vi "Curva suporte.vi"(8 "error in (no error)":errorcluster, 11 "Dados SP":T1={"Condutor"={"Pc (N/m)"=0.0, "Mod.Young (N/m²)"=0.0, "Dil.Term.c (m/°C)"=0.0, "Área  (m²)"=0.0, "Tração EDS (N)"=0.0, "Tração Torig(N)"=0.0, "Tração Talta (N)"=0.0}, "Suporte"={"Ps (N/m)"=0.0, "Es (N/m²)"=0.0, "DTc (1/°C)"=0.0, "Área sup (m²)"=0.0, "Tração EDS sup (N)"=0.0, "Tração AT sup (N)"=0.0, "Flecha sup AT (m)"=0.0}, "Projeto"={"Temp. EDS (°C)"=0.0, "Lim.original (°C)"=0.0, "Lim.extend. (°C)"=0.0, "N. cabo/fase"=1.0}, "Vetor de dados"={"Coor.X.esp"=[], "Coor.Y.Esp."=[], "Sub.vao X"=[], "Sub.vao Y"=[], "CoordY.sup"=[], "CoordX.sup"=[]}, "Subvão"={"N. Esp."=0.0, "F.lim (m)"=0.0, "Ext.calc"=0.0, "Ext.definido"=0.0, "Comp.cabo"=0.0, "Ext.55%"=0.0, "Tração sub\nAT (N)"=0.0, "Ext.sel."=0.0, "Flecha lim.\ncalc (m)"=0.0}, "Vão"={"Extensão (m)"=0.0, "Desnivel (m)"=0.0, "Ext.Lim sub (m)"=0.0, "Flecha à 60 °C"=0.0}} {"Projeto"."N. cabo/fase" min=1.0 max=8.0 step=1.0 format="%#_1f"}) -> (0 "error out":errorcluster, 3 "Dados SP Out":T1={"Condutor"={"Pc (N/m)"=0.0, "Mod.Young (N/m²)"=0.0, "Dil.Term.c (m/°C)"=0.0, "Área  (m²)"=0.0, "Tração EDS (N)"=0.0, "Tração Torig(N)"=0.0, "Tração Talta (N)"=0.0}, "Suporte"={"Ps (N/m)"=0.0, "Es (N/m²)"=0.0, "DTc (1/°C)"=0.0, "Área sup (m²)"=0.0, "Tração EDS sup (N)"=0.0, "Tração AT sup (N)"=0.0, "Flecha sup AT (m)"=0.0}, "Projeto"={"Temp. EDS (°C)"=0.0, "Lim.original (°C)"=0.0, "Lim.extend. (°C)"=0.0, "N. cabo/fase"=1.0}, "Vetor de dados"={"Coor.X.esp"=[], "Coor.Y.Esp."=[], "Sub.vao X"=[], "Sub.vao Y"=[], "CoordY.sup"=[], "CoordX.sup"=[]}, "Subvão"={"N. Esp."=0.0, "F.lim (m)"=0.0, "Ext.calc"=0.0, "Ext.definido"=0.0, "Comp.cabo"=0.0, "Ext.55%"=0.0, "Tração sub\nAT (N)"=0.0, "Ext.sel."=0.0, "Flecha lim.\ncalc (m)"=0.0}, "Vão"={"Extensão (m)"=0.0, "Desnivel (m)"=0.0, "Ext.Lim sub (m)"=0.0, "Flecha à 60 °C"=0.0}} {"Projeto"."N. cabo/fase" min=1.0 max=8.0 step=1.0 format="%#_1f"})   [LabVIEW 2020]
uses:
  controles/SP data.ctl
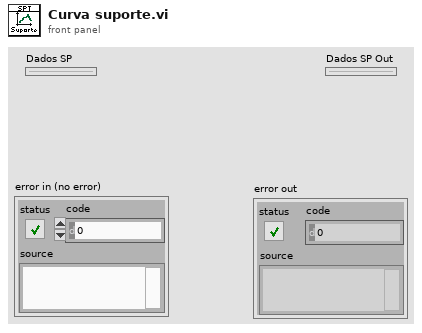
[diagram p1: front panel]
types:
  T1 = typedef "SP data.ctl" = cluster{"Condutor":cluster{"Pc (N/m)":dbl, "Mod.Young (N/m²)":dbl, "Dil.Term.c (m/°C)":dbl, "Área  (m²)":dbl, "Tração EDS (N)":dbl, "Tração Torig(N)":dbl, "Tração Talta (N)":dbl}, "Suporte":cluster{"Ps (N/m)":dbl, "Es (N/m²)":dbl, "DTc (1/°C)":dbl, "Área sup (m²)":dbl, "Tração EDS sup (N)":dbl, "Tração AT sup (N)":dbl, "Flecha sup AT (m)":dbl}, "Projeto":cluster{"Temp. EDS (°C)":dbl, "Lim.original (°C)":dbl, "Lim.extend. (°C)":dbl, "N. cabo/fase":dbl}, "Vetor de dados":cluster{"Coor.X.esp":dbl[], "Coor.Y.Esp.":dbl[], "Sub.vao X":dbl[], "Sub.vao Y":dbl[], "CoordY.sup":dbl[], "CoordX.sup":dbl[]}, "Subvão":cluster{"N. Esp.":dbl, "F.lim (m)":dbl, "Ext.calc":dbl, "Ext.definido":dbl, "Comp.cabo":dbl, "Ext.55%":dbl, "Tração sub\nAT (N)":dbl, "Ext.sel.":dbl, "Flecha lim.\ncalc (m)":dbl}, "Vão":cluster{"Extensão (m)":dbl, "Desnivel (m)":dbl, "Ext.Lim sub (m)":dbl, "Flecha à 60 °C":dbl}}
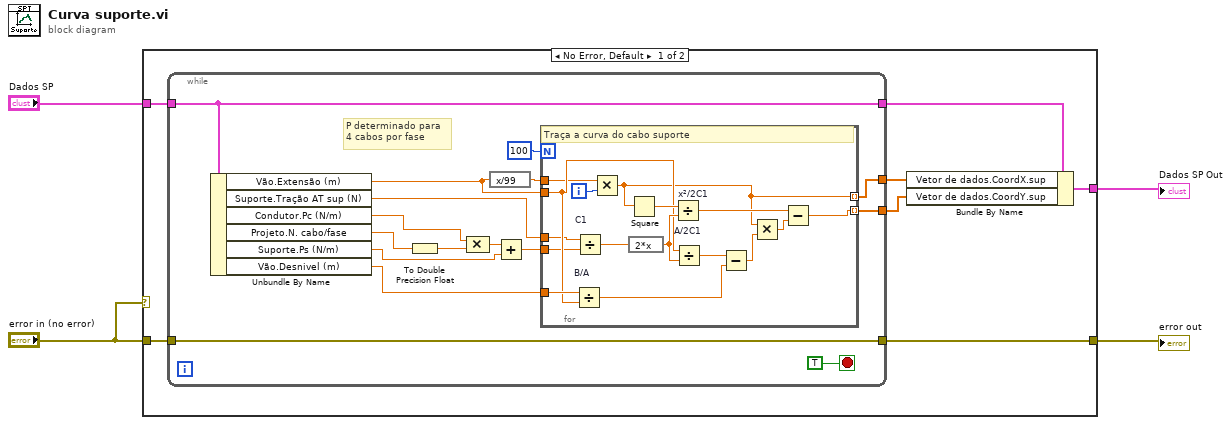
[diagram p0: block diagram]
diagram:
  n1 = case shown="No Error, Default" "error in (no error)" {
    tunnel: "Dados SP" -> [w11 w45]
    tunnel: "error in (no error)" -> [w10 w44]
    tunnel: [w9 w44] -> w3
    tunnel: [w5 w45] -> w2
    frame No Error {
      n2 = while {
        tunnel: [w26] -> w6
        tunnel: [w25] -> w7
        tunnel: w11 -> [w17]
        tunnel: w10 -> [w18]
        tunnel: [w18] -> w9
        tunnel: [w17] -> w8
        stop <- TRUE stop-if-true
        # "P determinado para\n4 cabos por fase"
        n3 = Unbundle By Name(w17) -> ("Vão.Extensão (m)"=w22:dbl, "Suporte.Tração AT sup (N)"=w21:dbl, "Condutor.Pc (N/m)"=w14:dbl, "Projeto.N. cabo/fase"=w13:dbl, "Suporte.Ps (N/m)"=w20:dbl, "Vão.Desnivel (m)"=w19:dbl)
        n4 = To Double Precision Float(number=w13) -> (double precision float=w15:dbl)
        n5 = Compound Arithmetic op=MULTIPLY(w14, w15) -> (w12:dbl)
        n6 = expression code="x/99"(w22) -> (w24:dbl)
        n7 = Add(x=w12, y=w20) -> (x+y=w27:dbl)
        n8 = for {
          N: 100 -> [_]
          tunnel: w19 -> [w35]
          tunnel: w22 -> [w34]
          tunnel: w27 -> [w33]
          tunnel: w24 -> [w32]
          tunnel: [w29] -> w25 mode=indexing
          tunnel: [w28] -> w26 mode=indexing
          tunnel: w21 -> [w30]
          i -> [w31]
          # "Traça a curva do cabo suporte"
          n9 = Divide "B/A"(x=w35, y=w34) -> (x/y=w41:dbl)
          n10 = Divide "C1"(x=w30, y=w33) -> (x/y=w43:dbl)
          n11 = Multiply(x=w32, y=w31) -> (x*y=w29:dbl)
          n12 = Square(x=w29) -> (x^2=w37:dbl)
          n13 = expression code="2*x"(w43) -> (w38:dbl)
          n14 = Divide "x²/2C1"(x=w37, y=w38) -> (x/y=w36:dbl)
          n15 = Divide "A/2C1"(x=w34, y=w38) -> (x/y=w42:dbl)
          n16 = Subtract(x=w42, y=w41) -> (x-y=w40:dbl)
          n17 = Multiply(x=w29, y=w40) -> (x*y=w39:dbl)
          n18 = Subtract(x=w36, y=w39) -> (x-y=w28:dbl)
        }
      }
      n19 = Bundle By Name(cluster=w8, "Vetor de dados.CoordX.sup"=w7, "Vetor de dados.CoordY.sup"=w6) -> (w5:T1)
    }
    frame Error {
    }
  }
  "error out" <- w3
  "Dados SP Out" <- w2
